vi "GB_Test.vi"(8 "Error In":errorcluster, 10 "PORT":string, 11 "Limit":string) -> (0 "error out":errorcluster, 2 "Result":bool, 3 "Data":string)   [LabVIEW 2013]
uses:
  MainProgram/Control/Buffer.vi
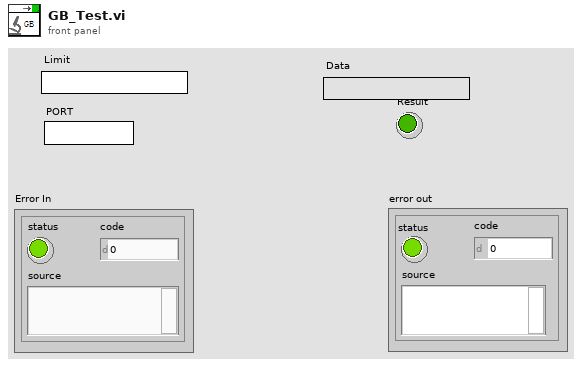
[diagram p1: front panel]
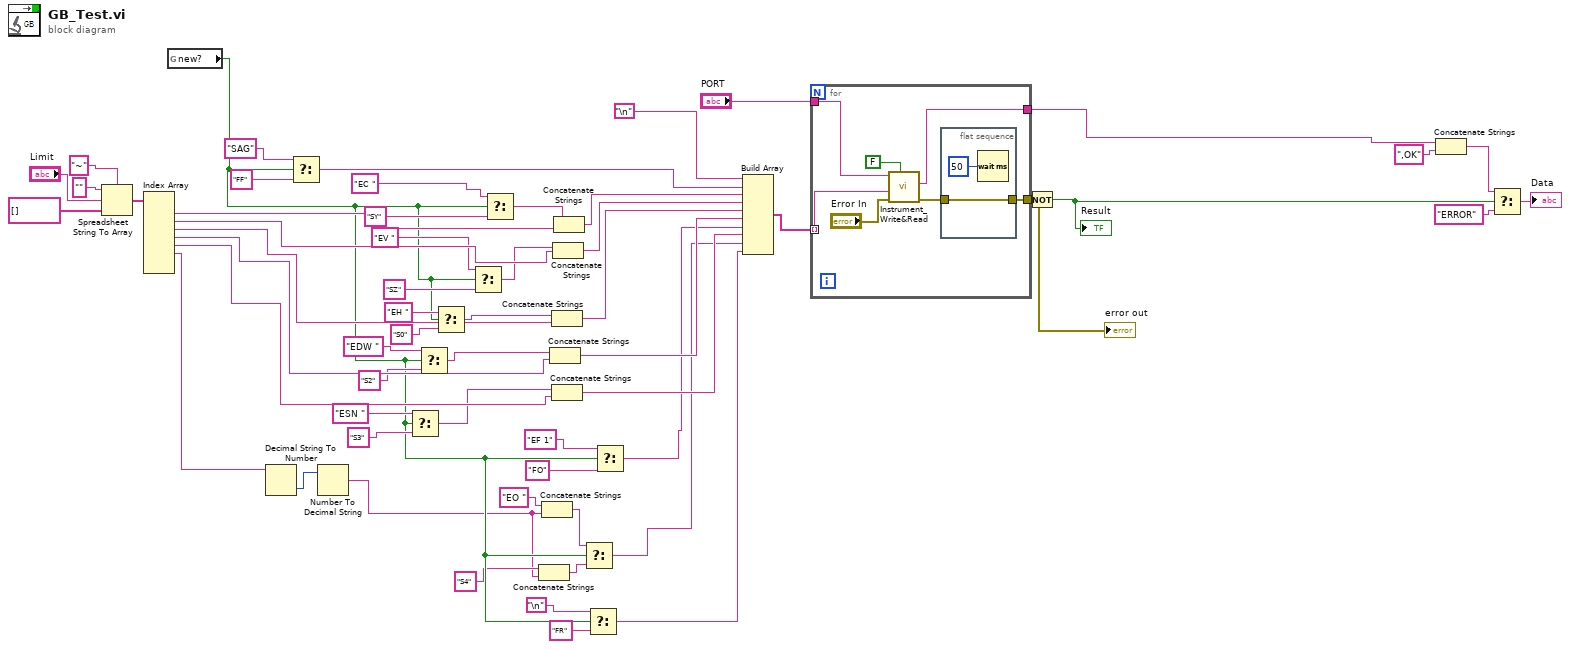
[diagram p0: block diagram]
diagram:
  n1 = Spreadsheet String To Array(delimiter (Tab)="~", format string="", spreadsheet string="Limit", array type (2D Dbl)=string[] []) -> (array=w52:string[])
  n2 = Index Array(array=w52) -> (element #1=w41:string, element #2=w40:string, element #3=w39:string, element #4=w38:string, element #5=w35:string, element #6=w7:string)  [unwired: 8 in, 2 out]
  n3 = global read "Buffer.vi" "new?"() -> (w11:bool)
  n4 = Decimal String To Number(string=w7) -> (number=w1:i32)  [unwired: 2 in, 1 out]
  n5 = Select(t="SAG" ("format string"), s=w11, f="FF" ("format string")) -> (s? t:f=w32:string)
  n6 = Number To Decimal String(number=w1) -> (decimal integer string=w2:string)  [unwired: 1 in]
  n7 = Select(t="ESN " ("element"), s=w11, f="S3" ("element")) -> (s? t:f=w17:string)
  n8 = Select(t="EDW " ("string"), s=w11, f="S2" ("string")) -> (s? t:f=w20:string)
  n9 = Select(t="EH " ("string"), s=w11, f="S0" ("string")) -> (s? t:f=w23:string)
  n10 = Select(t="EV " ("string"), s=w11, f="SZ" ("string")) -> (s? t:f=w26:string)
  n11 = Select(t="EC " ("string"), s=w11, f="SY" ("string")) -> (s? t:f=w29:string)
  n12 = Concatenate Strings("S4" ("element"), w2) -> (w3:string)
  n13 = Concatenate Strings("EO " ("element"), w2) -> (w5:string)
  n14 = Concatenate Strings(w20, w38) -> (w36:string)
  n15 = Concatenate Strings(w23, w39) -> (w43:string)
  n16 = Concatenate Strings(w17, w35) -> (w34:string)
  n17 = Concatenate Strings(w26, w40) -> (w44:string)
  n18 = Concatenate Strings(w29, w41) -> (w45:string)
  n19 = Select(t=w5, s=w11, f=w3) -> (s? t:f=w12:string)
  n20 = Select(t="\n", s=w11, f="FR") -> (s? t:f=w9:string)
  n21 = Select(t="EF 1" ("element"), s=w11, f="FO" ("element")) -> (s? t:f=w14:string)
  n22 = Build Array("\n", w32, w45, w44, w43, w36, w14, w34, w12, w9) -> (w42:string[])
  n23 = for {
    tunnel: [w59] -> w50
    tunnel: "PORT" -> [w63]
    tunnel: [w62] -> w46
    tunnel: w42 -> [w61] mode=indexing
    n24 = call "Instrument_Write&Read.vi"("Read?"=FALSE, "Error In"="Error In", "CMD"=w61, "PORT"=w63) -> ("Error Out"=w60:errorcluster, "read buffer"=w62:string)  [unwired: 6 in]
    n25 = flat-sequence {
      tunnel: w60 -> [w67]
      tunnel: [w67] -> w59
      frame #0 {
        n26 = Wait (ms)(milliseconds to wait=u32 50) -> ()  [unwired: 1 out]
      }
    }
  }
  "error out" <- w50
  n27 = Not(x=w50) -> (.not. x?=w56:bool)
  "Result" <- w56
  n28 = Concatenate Strings(w46, ",OK") -> (w48:string)
  n29 = Select(t=w48, s=w56, f="ERROR") -> (s? t:f=→"Data":string)
